vi "Measurement UI.vi"() -> ()   [LabVIEW 2021, in "Crosstalk_Class D Amplifier.lvlib"]
uses:
  Crosstalk_Class D Amplifier.lvlib
panel:
  in  "Graphs":enum32{"Frequency Domain", "Time Domain"}(tab)
  out "frequency domain":T1(graph)
  out "time domain":waveform(dbl)[](graph)
  out "meas table":string[][](table)
  out "output power (W)":dbl
  out "wfm_interferrer - data":dbl[](array[numeric])
  out "fft_interferrer - data":dbl[](array[numeric])
  in  "Configuration tab":enum32{"Protocol", "Measurement"}(tab)
  in  "master clock channel list":string caption="Master Clock Channel"
  in  "digital channel list":string caption="Digital Audio Channel"
  in  "logic level":enum32{"3.3 V", "1.8 V", "1.2 V"}(ring) caption="Logic level"
  in  "master clock rate":dbl=12288000.0 caption="Master clock rate" format="%#_6pHz"
  out "Bit clock rate":dbl=3072000.0 format="%#_6pHz"
  in  "number of channels":u8=2 caption="Number of channels"
  in  "TDM":bool
  in  "RJ":bool
  in  "LJ":bool
  in  "I2S":bool
  in  "bit clock edge sync":enum32{"Rising", "Falling"}(ring)=enum."Falling" caption="Bit clock edge sync"
  in  "frame clock rate":dbl=48000.0 caption="Frame clock rate" format="%#_6pHz"
  in  "data justification":enum32{"Left Justified", "Right Justified"}(ring) caption="Data justification"
  in  "endianness":enum32{"MSB First", "LSB First"}(ring) caption="Endianness"
  in  "bit depth":u8=24 caption="Bit depth"
  in  "channel length":u16=32 caption="Channel length"
  in  "frame sync edge for channel 0":enum32{"Rising", "Falling"}(ring)=enum."Falling" caption="Frame sync edge for Channel 0"
  in  "min settling cycles":u32 caption="Minimum settling cycles"
  in  "min settling time (s)":dbl=0.1 caption="Minimum settling time" format="%#_6ps"
  in  "min measurement cycles":u32 caption="Minimum measurement cycles"
  in  "min measurement time (s)":dbl=0.1 caption="Minimum measurement time" format="%#_6ps"
  in  "lowpass filter":T2(ring) caption="Lowpass filter"
  in  "highpass filter":enum32{"DC", "AC"}(ring) caption="Highpass filter"
  in  "output power (W)":dbl=1.0 caption="Output power" format="%#_6p W"
  in  "output mode":enum16{"Level", "Power"}(ring) caption="Output mode"
  in  "load impedance":dbl=-1.0 caption="Load impedance" format="%#_6p Ohms"
  in  "acq channel - interferrer":string caption="Interferrer channel resource"
  in  "acq channel - victim":string caption="Victim channel resource"
  in  "digital audio interferrer channel":i32=1000 caption="Interferrer channel"
  in  "output range (pk-pk)":dbl=15.0 caption="Output range" format="%.3p Vpk-pk"
  in  "signal frequency":dbl=1000.0 caption="Frequency" format="%#_6pHz"
  in  "output level (dB)":dbl=-1.0 caption="Output level" format="%#_6p dBFS"
  in  "acq sampling rate":dbl=51200.0 caption="Sample rate" format="%#.6pHz"
  in  "channel 0 offset":u32=1
  out "fft_victim - data":dbl[](array[numeric])
  out "fft - df":dbl
  out "fft - f0":dbl
  out "wfm_victim - data":dbl[](array[numeric])
  out "wfm - dt":dbl
  out "crosstalk (dB)":dbl
  out "measured frequency (Hz)":dbl
  out "Channel name":string
  in  "acq channel":string="PXI1Slot4/ai0"
  in  "signal phase":dbl caption="phase"
  # "hidden controls - used to sync with MeasLink"
  # "hidden indicators"
  # "Protocols"
  # "Audio Protocol"
  # "Clock Settings"
  # "Signal Level"
  # "Harware Resource"
  # "Filters"
  # "Output"
  # "Acquisition"
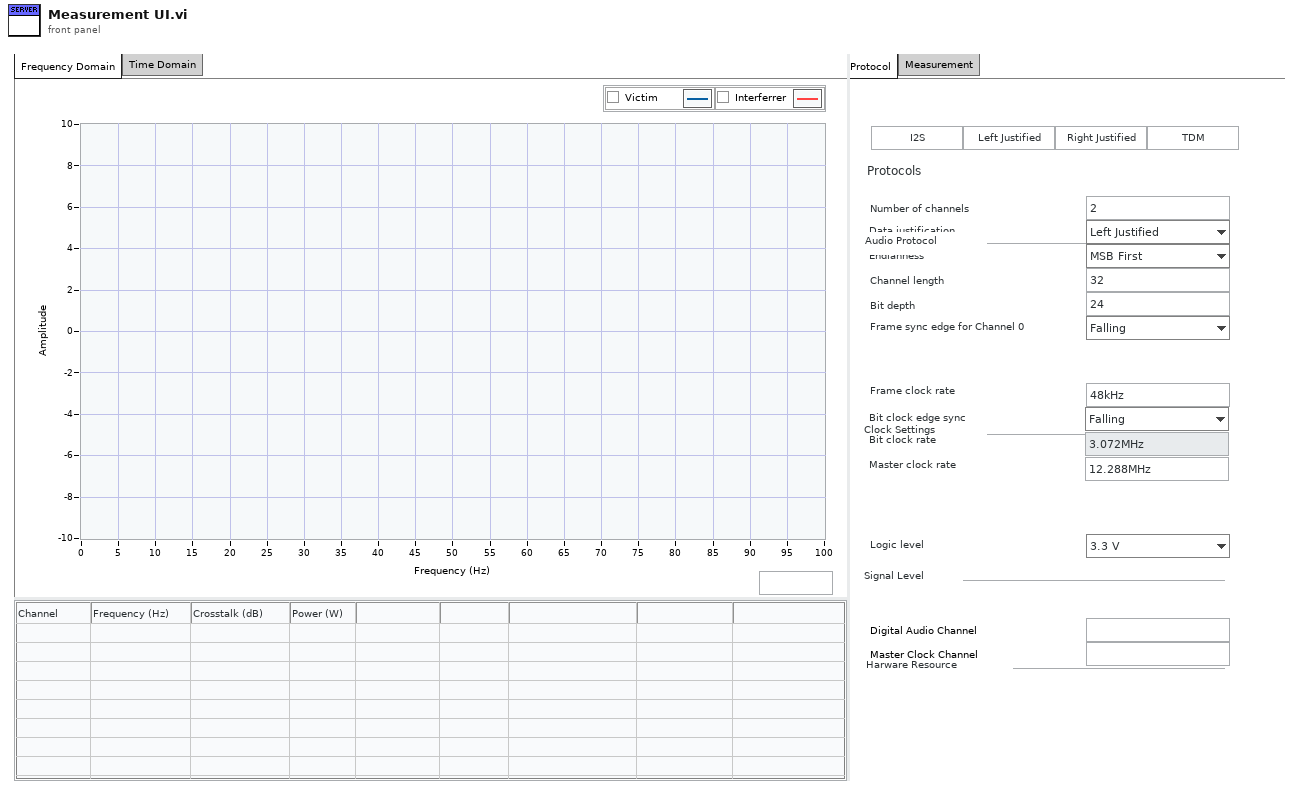
[diagram p1: front panel]
types:
  T1 = cluster{"fft - f0":dbl, "fft - df":dbl, "fft_interferrer - data":dbl[]}[]
  T2 = enum32{"No filter", "AES17 20kHz", "AES17 40kHz"}
  T3 = cluster{"fft - f0":dbl, "fft - df":dbl, "fft_victim - data":dbl[]}
  T4 = cluster{"fft - f0":dbl, "fft - df":dbl, "fft_interferrer - data":dbl[]}
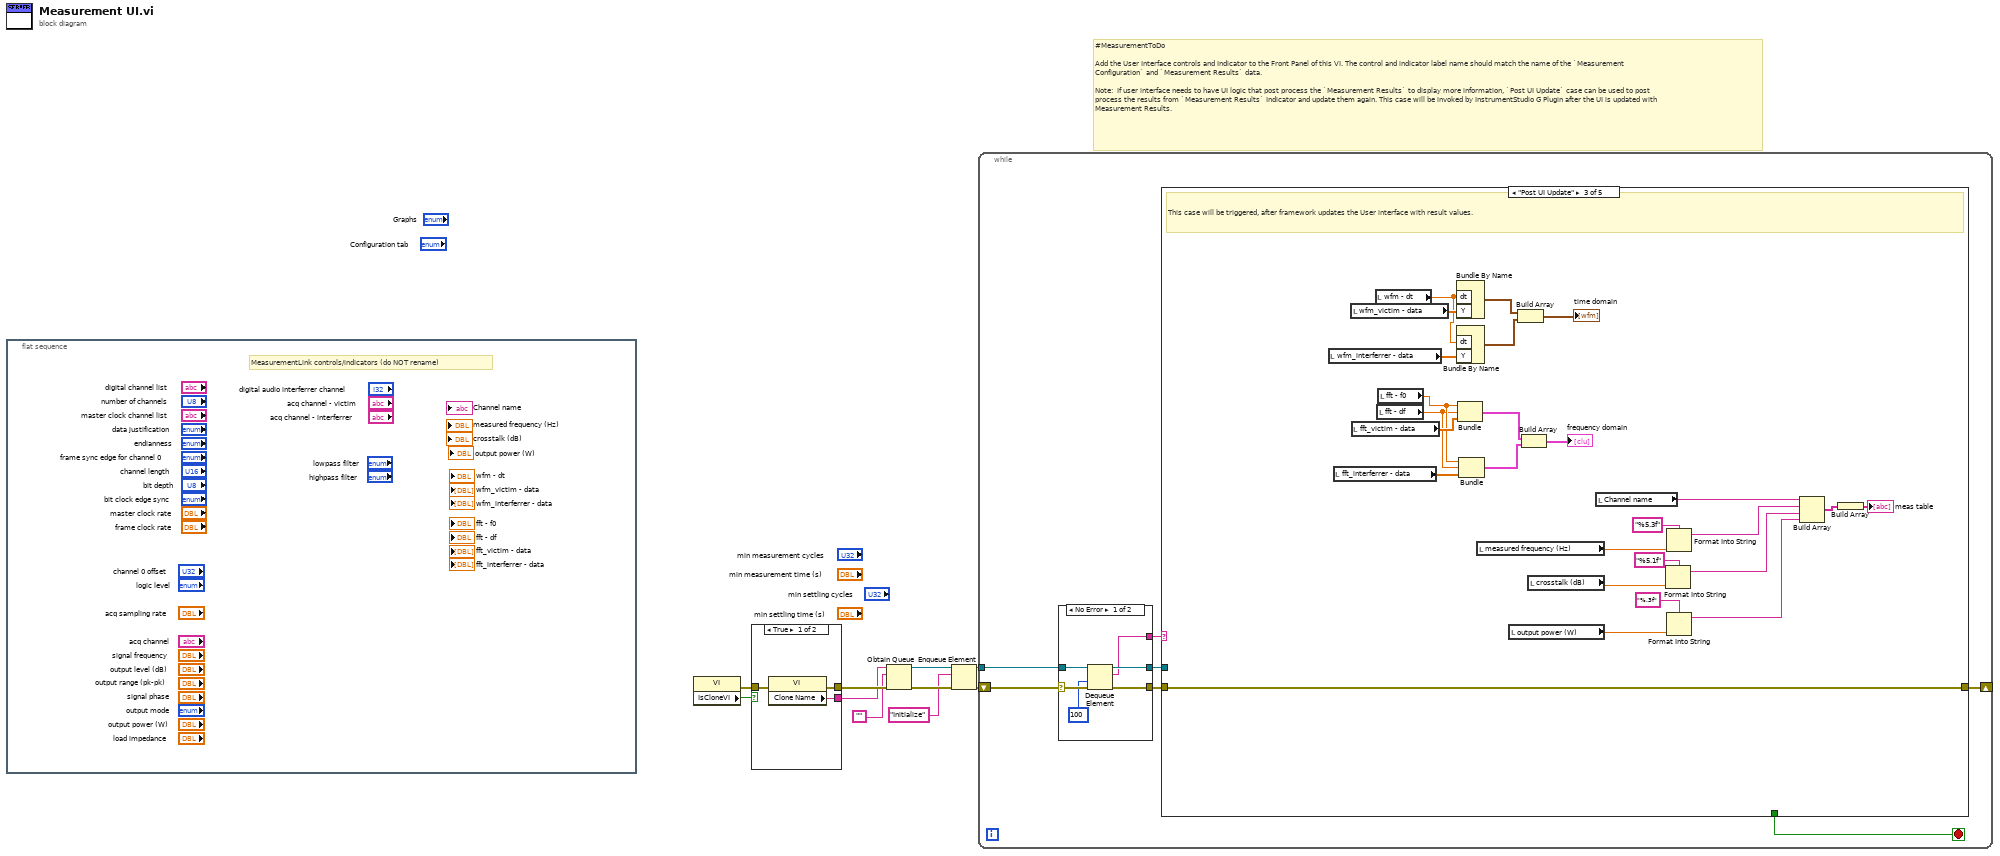
[diagram p0: block diagram]
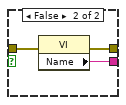
[diagram p2: hidden frame]
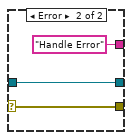
[diagram p3: hidden frame]
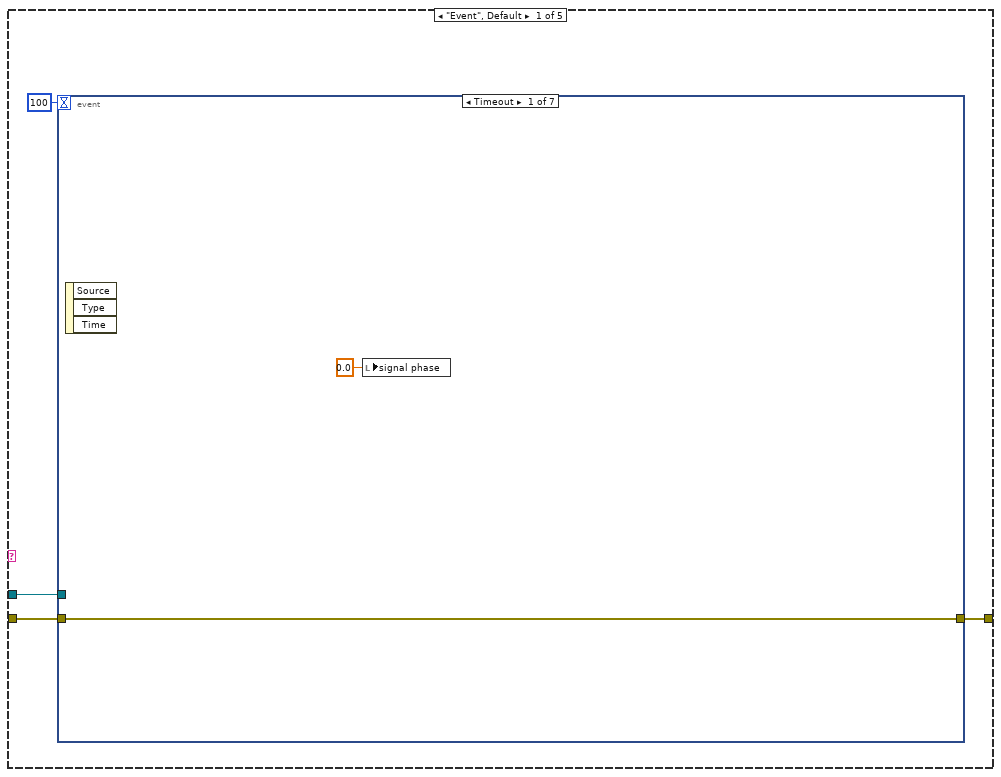
[diagram p4: hidden frame]
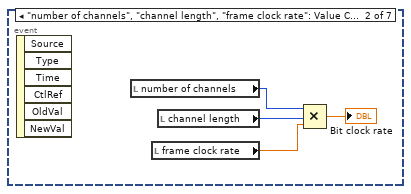
[diagram p5: hidden frame]
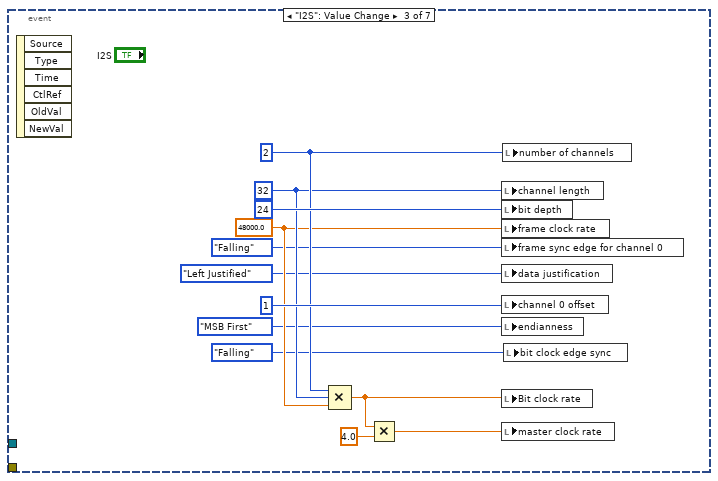
[diagram p6: hidden frame]
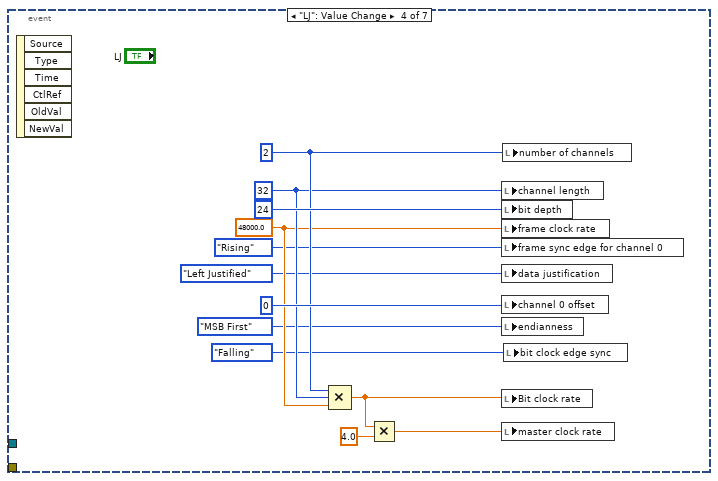
[diagram p7: hidden frame]
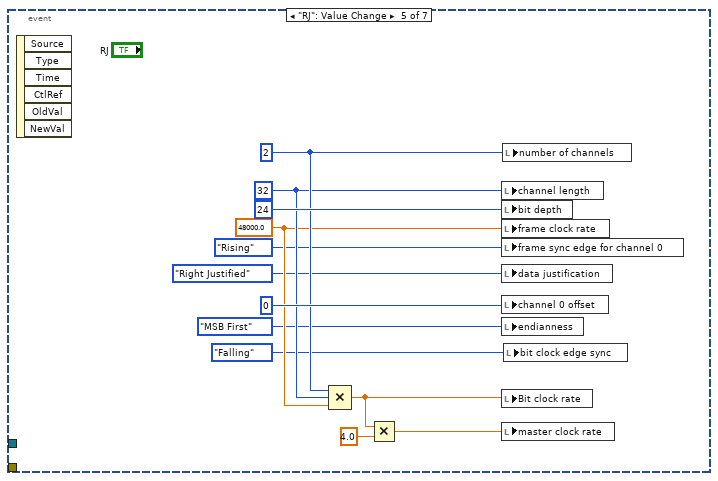
[diagram p8: hidden frame]
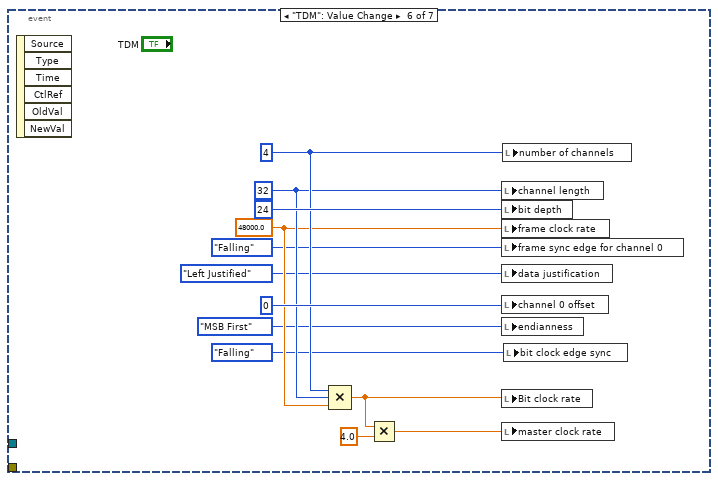
[diagram p9: hidden frame]
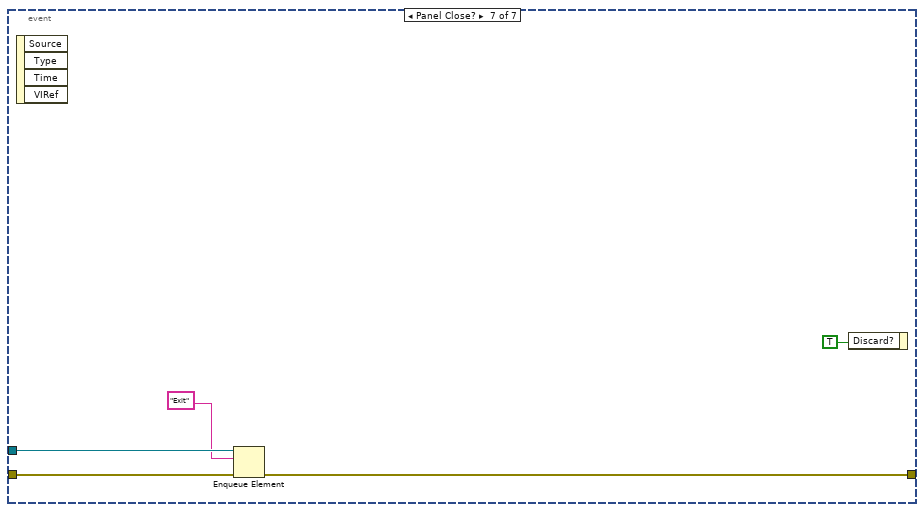
[diagram p10: hidden frame]
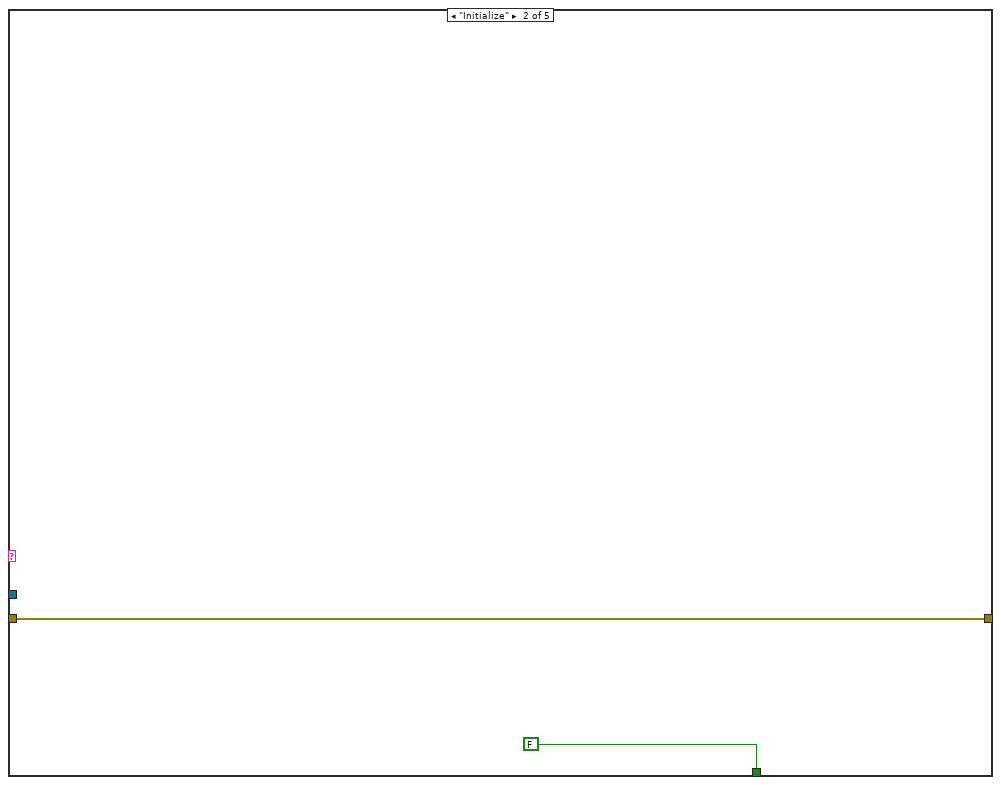
[diagram p11: hidden frame]
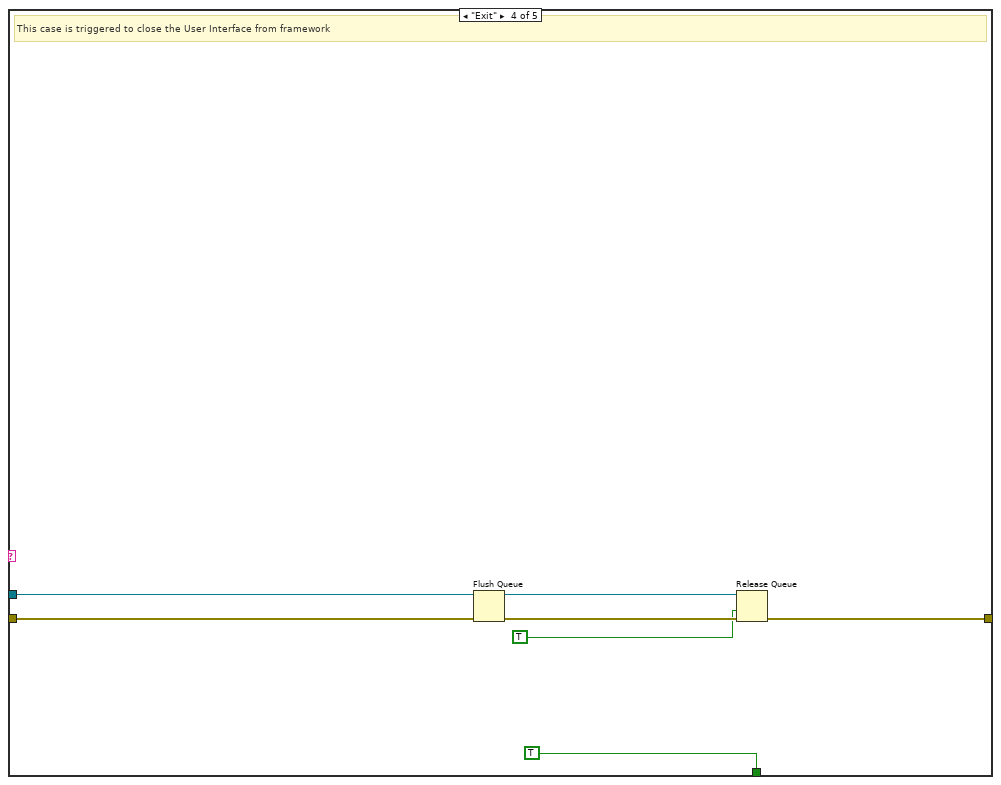
[diagram p12: hidden frame]
diagram:
  # "#MeasurementToDo  \n\nAdd the User Interface controls and Indicator to the Front Panel of this VI. The control and indicator label name should match the name of the `Measurement Configuration` and `Measurement Results` data.\n\nNote:  If user interface needs to have UI logic that post process the `Measurement Results` to display more information, `Post UI Update` case can be used to post process the results from `Measurement Results` Indicator and update them again. This case will be invoked by InstrumentStudio G Plugin after the UI is updated with Measurement Results."
  n1 = flat-sequence {
    frame #0 {
      # "MeasurementLink controls/indicators (do NOT rename)"
    }
  }
  n2 = property class="VI"() -> (error out=w1:errorcluster, "IsCloneVI"=w2:bool)  [unwired: 2 in, 1 out]
  n3 = case shown="True" w2 {
    tunnel: [w13 w16] -> w10
    tunnel: [w12 w15] -> w9
    tunnel: w1 -> [w11 w14]
    frame True {
      n4 = property class="VI"(error in=w11) -> (error out=w13:errorcluster, "Clone Name"=w12:string)  [unwired: 1 in, 1 out]
    }
    frame False {
      n5 = property class="VI"(error in=w14) -> (error out=w16:errorcluster, "Name"=w15:string)  [unwired: 1 in, 1 out]
    }
  }
  n6 = Obtain Queue(name (unnamed)=w9, element data type="", error in (no error)=w10) -> (queue out=w6:refnum<queue>, error out=w8:errorcluster)  [unwired: 2 in, 1 out]
  n7 = Enqueue Element(queue=w6, element="Initialize", error in (no error)=w8) -> (queue out=w5:refnum<queue>, error out=w7:errorcluster)  [unwired: 1 in, 1 out]
  n8 = while {
    shift-right: [w18] -> _
    shift-left: w7 -> [w23]
    tunnel: w5 -> [w21]
    stop <- w17 stop-if-true
    n9 = case shown="No Error" w23 {
      selector: w23 -> [w29 w32]
      tunnel: [w28 w32] -> w22
      tunnel: w21 -> [w27 w31]
      tunnel: [w26 w31] -> w20
      tunnel: [w25 "Handle Error"] -> w19
      frame No Error {
        n10 = Dequeue Element(queue=w27, timeout in ms (-1)=100, error in (no error)=w29) -> (queue out=w26:refnum<queue>, element=w25:string, error out=w28:errorcluster)  [unwired: 1 out]
      }
      frame Error {
      }
    }
    n11 = case shown="\"Post UI Update\"" w19 {
      tunnel: w22 -> [w35 w97 w123 w130 w131]
      tunnel: w20 -> [w33 _ _ w128 _]
      tunnel: [w36 w97 w123 w125 w131] -> w18
      tunnel: [_ FALSE _ TRUE _] -> w17
      frame "Event", Default {
        n12 = event shown="[0] Timeout" {
          selector: _ -> [_ _ _ _ _ _ _]
          dyn-events: _ -> [_ _ _ _ _ _ _]
          timeout: 100 -> [_ _ _ _ _ _ _]
          tunnel: [w38 _ _ _ _ _ w93] -> w36
          tunnel: w35 -> [w38 _ _ _ _ _ w94]
          tunnel: w33 -> [_ _ _ _ _ _ w92]
          event Timeout {
            n13 = event-data() -> ()  [unwired: 1 in, 3 out]
            n14 = local write "signal phase"(0.0 ("signal phase")) -> ()
          }
          event "number of channels", "channel length", "frame clock rate": Value Change {
            n15 = event-data() -> ()  [unwired: 1 in, 6 out]
            n16 = local read "number of channels"() -> (w42:u8)
            n17 = local read "frame clock rate"() -> (w40:dbl)
            n18 = local read "channel length"() -> (w41:u16)
            n19 = Compound Arithmetic op=MULTIPLY(w42, w41, w40) -> (→"Bit clock rate":dbl)
          }
          event "I2S": Value Change {
            w50 = 48000.0 ("Frame Clock Rate")
            w51 = u32 32 ("Channel Length")
            w52 = u32 2 ("Number of Channels")
            n20 = event-data() -> ()  [unwired: 1 in, 6 out]
            n21 = Compound Arithmetic op=MULTIPLY(w52, w51, w50) -> (w49:dbl)
            n22 = Multiply(x=w49, y=4.0) -> (x*y=w48:dbl)
            n23 = local write "channel length"(w51) -> ()
            n24 = local write "bit depth"(u32 24 ("Bit Depth")) -> ()
            n25 = local write "frame clock rate"(w50) -> ()
            n26 = local write "frame sync edge for channel 0"(enum32{"Rising", "Falling"}."Falling" ("bit clock edge sync")) -> ()
            n27 = local write "data justification"(enum32{"Left Justified", "Right Justified"}."Left Justified" ("data justification")) -> ()
            n28 = local write "channel 0 offset"(u32 1 ("Channel 0 Offset")) -> ()
            n29 = local write "endianness"(enum32{"MSB First", "LSB First"}."MSB First" ("endianness")) -> ()
            n30 = local write "Bit clock rate"(w49) -> ()
            n31 = local write "master clock rate"(w48) -> ()
            n32 = local write "number of channels"(w52) -> ()
            n33 = local write "bit clock edge sync"(enum32{"Rising", "Falling"}."Falling" ("frame sync edge for channel 0")) -> ()
          }
          event "LJ": Value Change {
            w62 = 48000.0 ("Frame Clock Rate")
            w63 = u32 32 ("Channel Length")
            w64 = u32 2 ("Number of Channels")
            n34 = event-data() -> ()  [unwired: 1 in, 6 out]
            n35 = Compound Arithmetic op=MULTIPLY(w64, w63, w62) -> (w61:dbl)
            n36 = Multiply(x=w61, y=4.0) -> (x*y=w60:dbl)
            n37 = local write "channel length"(w63) -> ()
            n38 = local write "bit depth"(u32 24 ("Bit Depth")) -> ()
            n39 = local write "frame clock rate"(w62) -> ()
            n40 = local write "frame sync edge for channel 0"(enum32{"Rising", "Falling"}."Rising" ("bit clock edge sync")) -> ()
            n41 = local write "data justification"(enum32{"Left Justified", "Right Justified"}."Left Justified" ("data justification")) -> ()
            n42 = local write "channel 0 offset"(u32 0 ("Channel 0 Offset")) -> ()
            n43 = local write "endianness"(enum32{"MSB First", "LSB First"}."MSB First" ("endianness")) -> ()
            n44 = local write "Bit clock rate"(w61) -> ()
            n45 = local write "master clock rate"(w60) -> ()
            n46 = local write "number of channels"(w64) -> ()
            n47 = local write "bit clock edge sync"(enum32{"Rising", "Falling"}."Falling" ("frame sync edge for channel 0")) -> ()
          }
          event "RJ": Value Change {
            w74 = 48000.0 ("Frame Clock Rate")
            w75 = u32 32 ("Channel Length")
            w76 = u32 2 ("Number of Channels")
            n48 = event-data() -> ()  [unwired: 1 in, 6 out]
            n49 = Compound Arithmetic op=MULTIPLY(w76, w75, w74) -> (w73:dbl)
            n50 = Multiply(x=w73, y=4.0) -> (x*y=w72:dbl)
            n51 = local write "channel length"(w75) -> ()
            n52 = local write "bit depth"(u32 24 ("Bit Depth")) -> ()
            n53 = local write "frame clock rate"(w74) -> ()
            n54 = local write "frame sync edge for channel 0"(enum32{"Rising", "Falling"}."Rising" ("bit clock edge sync")) -> ()
            n55 = local write "data justification"(enum32{"Left Justified", "Right Justified"}."Right Justified" ("data justification")) -> ()
            n56 = local write "channel 0 offset"(u32 0 ("Channel 0 Offset")) -> ()
            n57 = local write "endianness"(enum32{"MSB First", "LSB First"}."MSB First" ("endianness")) -> ()
            n58 = local write "Bit clock rate"(w73) -> ()
            n59 = local write "master clock rate"(w72) -> ()
            n60 = local write "number of channels"(w76) -> ()
            n61 = local write "bit clock edge sync"(enum32{"Rising", "Falling"}."Falling" ("frame sync edge for channel 0")) -> ()
          }
          event "TDM": Value Change {
            w86 = 48000.0 ("Frame Clock Rate")
            w87 = u32 32 ("Channel Length")
            w88 = u32 4 ("Number of Channels")
            n62 = event-data() -> ()  [unwired: 1 in, 6 out]
            n63 = Compound Arithmetic op=MULTIPLY(w88, w87, w86) -> (w85:dbl)
            n64 = Multiply(x=w85, y=4.0) -> (x*y=w84:dbl)
            n65 = local write "channel length"(w87) -> ()
            n66 = local write "bit depth"(u32 24 ("Bit Depth")) -> ()
            n67 = local write "frame clock rate"(w86) -> ()
            n68 = local write "frame sync edge for channel 0"(enum32{"Rising", "Falling"}."Falling" ("bit clock edge sync")) -> ()
            n69 = local write "data justification"(enum32{"Left Justified", "Right Justified"}."Left Justified" ("data justification")) -> ()
            n70 = local write "channel 0 offset"(u32 0 ("Channel 0 Offset")) -> ()
            n71 = local write "endianness"(enum32{"MSB First", "LSB First"}."MSB First" ("endianness")) -> ()
            n72 = local write "Bit clock rate"(w85) -> ()
            n73 = local write "master clock rate"(w84) -> ()
            n74 = local write "number of channels"(w88) -> ()
            n75 = local write "bit clock edge sync"(enum32{"Rising", "Falling"}."Falling" ("frame sync edge for channel 0")) -> ()
          }
          event Panel Close? {
            n76 = event-data() -> ()  [unwired: 1 in, 4 out]
            n77 = Enqueue Element(queue=w92, element="Exit", error in (no error)=w94) -> (error out=w93:errorcluster)  [unwired: 1 in, 2 out]
            n78 = event-data("Discard?"=TRUE) -> ()  [unwired: 1 in, 1 out]
          }
        }
      }
      frame "Initialize" {
      }
      frame "Post UI Update" {
        # "This case will be triggered, after framework updates the User interface with result values."
        n79 = local read "wfm_interferrer - data"() -> (w110:dbl[])
        n80 = local read "fft_interferrer - data"() -> (w104:dbl[])
        n81 = local read "wfm_victim - data"() -> (w122:dbl[])
        n82 = local read "fft_victim - data"() -> (w121:dbl[])
        n83 = local read "wfm - dt"() -> (w111:dbl)
        n84 = local read "fft - df"() -> (w105:dbl)
        n85 = local read "fft - f0"() -> (w106:dbl)
        n86 = Bundle By Name("dt"=w111, "Y"=w122) -> (w109:waveform(dbl))  [unwired: 1 in]
        n87 = Bundle By Name("dt"=w111, "Y"=w110) -> (w108:waveform(dbl))  [unwired: 1 in]
        n88 = Bundle("fft - f0"=w106, "fft - df"=w105, "fft_victim - data"=w121) -> (w103:T3)  [unwired: 1 in]
        n89 = Bundle("fft - f0"=w106, "fft - df"=w105, "fft_interferrer - data"=w104) -> (w102:T4)  [unwired: 1 in]
        n90 = local read "measured frequency (Hz)"() -> (w112:dbl)
        n91 = local read "output power (W)"() -> (w98:dbl)
        n92 = Build Array(w109, w108) -> (→"time domain":waveform(dbl)[])
        n93 = Build Array(w103, w102) -> (→"frequency domain":T1)
        n94 = local read "crosstalk (dB)"() -> (w113:dbl)
        n95 = local read "Channel name"() -> (w114:string)
        n96 = Format Into String(format string="%5.1f" ("initial string"), w113) -> (resulting string=w118:string)  [unwired: 2 in, 1 out]
        n97 = Format Into String(format string="%5.3f" ("initial string"), w112) -> (resulting string=w119:string)  [unwired: 2 in, 1 out]
        n98 = Format Into String(format string="%.3f" ("initial string"), w98) -> (resulting string=w100:string)  [unwired: 2 in, 1 out]
        n99 = Build Array(w114, w119, w118, w100) -> (w120:string[])
        n100 = Build Array(w120) -> (→"meas table":string[][])
      }
      frame "Exit" {
        # "This case is triggered to close the User Interface from framework"
        n101 = Flush Queue(queue=w128, error in (no error)=w130) -> (queue out=w127:refnum<queue>, error out=w126:errorcluster)  [unwired: 1 out]
        n102 = Release Queue(queue=w127, force destroy? (F)=TRUE, error in (no error)=w126) -> (error out=w125:errorcluster)  [unwired: 2 out]
      }
      frame "Handle Error" {
      }
    }
  }
